vi "RBF Graph Test.vi"() -> ()   [LabVIEW 2021]
panel:
  in  "Weights":dbl[](array[numeric])
  in  "RBF":cluster{"STD":dbl, "Number":i32}
  out "XY Graph":cluster{dbl[], dbl[]}[](graph)
  in  "x":cluster{"Number":i32, "x_0":dbl, "x_f":dbl}
  out "x":dbl[][](array[numeric])
  out "RBF Centers":dbl[][](array[numeric])
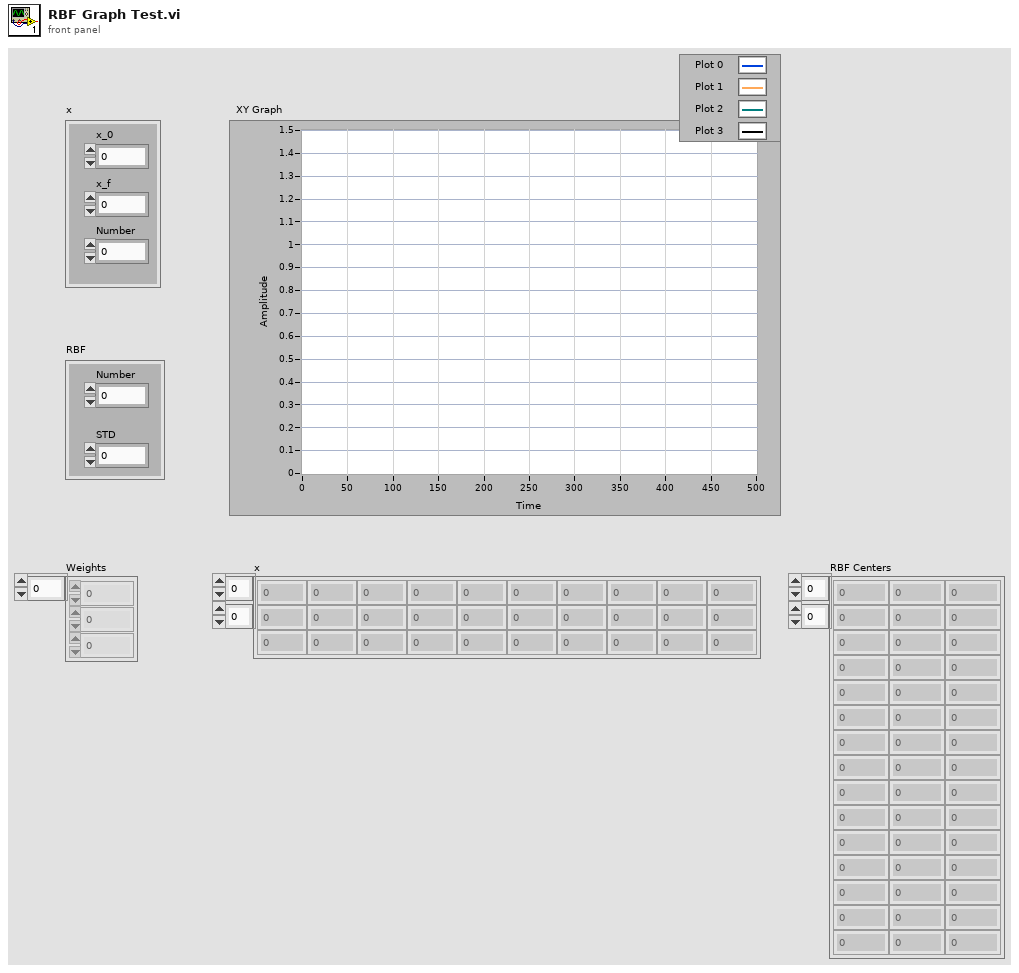
[diagram p1: front panel]
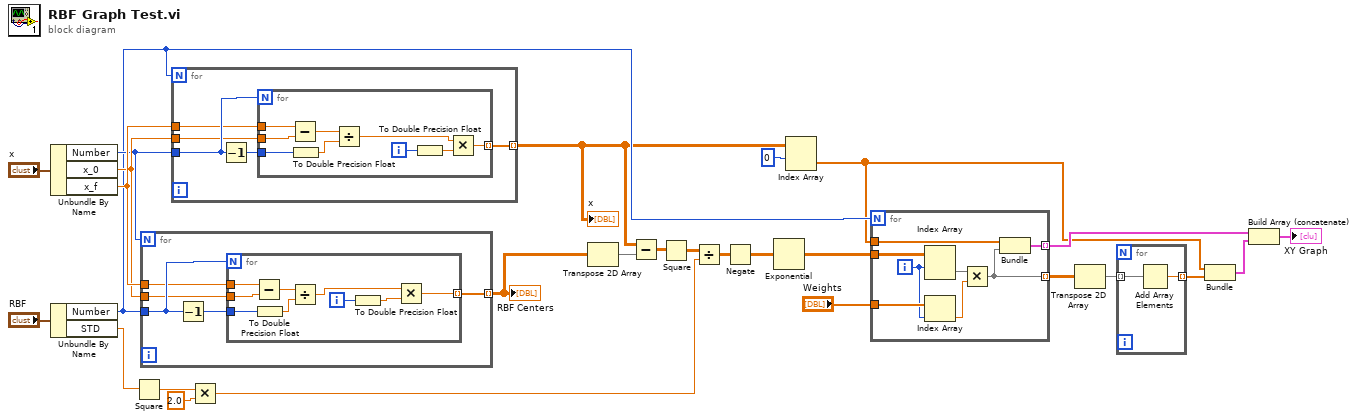
[diagram p0: block diagram]
diagram:
  n1 = Unbundle By Name("x") -> ("Number"=w15:i32, "x_0"=w17:dbl, "x_f"=w18:dbl)
  n2 = Unbundle By Name("RBF") -> ("Number"=w11:i32, "STD"=w16:dbl)
  n3 = Square(x=w16) -> (x^2=w25:dbl)
  n4 = for {
    N: w15 -> [_]
    tunnel: [w31] -> w13 mode=indexing
    tunnel: w11 -> [w30]
    tunnel: w18 -> [w29]
    tunnel: w17 -> [w28]
    n5 = Decrement(x=w30) -> (x-1=w32:i32)
    n6 = for {
      N: w30 -> [_]
      tunnel: w29 -> [w41]
      tunnel: w28 -> [w39]
      tunnel: [w40] -> w31 mode=indexing
      tunnel: w32 -> [w36]
      i -> [w34]
      n7 = Subtract(x=w41, y=w39) -> (x-y=w38:dbl)
      n8 = To Double Precision Float(number=w36) -> (double precision float=w35:dbl)
      n9 = Divide(x=w38, y=w35) -> (x/y=w37:dbl)
      n10 = To Double Precision Float(number=w34) -> (double precision float=w33:dbl)
      n11 = Multiply(x=w37, y=w33) -> (x*y=w40:dbl)
    }
  }
  "RBF Centers" <- w13
  n12 = for {
    N: w11 -> [_]
    tunnel: [w45] -> w5 mode=indexing
    tunnel: w15 -> [w44]
    tunnel: w18 -> [w43]
    tunnel: w17 -> [w42]
    n13 = Decrement(x=w44) -> (x-1=w46:i32)
    n14 = for {
      N: w44 -> [_]
      tunnel: w43 -> [w55]
      tunnel: w42 -> [w53]
      tunnel: [w54] -> w45 mode=indexing
      tunnel: w46 -> [w50]
      i -> [w47]
      n15 = Subtract(x=w55, y=w53) -> (x-y=w52:dbl)
      n16 = To Double Precision Float(number=w50) -> (double precision float=w49:dbl)
      n17 = Divide(x=w52, y=w49) -> (x/y=w51:dbl)
      n18 = To Double Precision Float(number=w47) -> (double precision float=w48:dbl)
      n19 = Multiply(x=w51, y=w48) -> (x*y=w54:dbl)
    }
  }
  "x" <- w5
  n20 = Multiply(x=w25, y=2.0) -> (x*y=w24:dbl)
  n21 = Transpose 2D Array(2D array=w13) -> (transposed array=w12:dbl[][])
  n22 = Subtract(x=w5, y=w12) -> (x-y=w27:dbl[][])
  n23 = Square(x=w27) -> (x^2=w23:dbl[][])
  n24 = Divide(x=w23, y=w24) -> (x/y=w22:dbl[][])
  n25 = Negate(x=w22) -> (-x=w21:dbl[][])
  n26 = Exponential(1:w21) -> (0:w2:dbl[][])
  n27 = Index Array(array=w5, index (row)=0) -> (element=w3:dbl[])  [unwired: 1 in]
  n28 = for {
    N: w11 -> [_]
    tunnel: w2 -> [w63]
    tunnel: [w62] -> w8 mode=indexing
    tunnel: "Weights" -> [w61]
    tunnel: w3 -> [w57]
    tunnel: [w56] -> w1 mode=indexing
    i -> [w60]
    n29 = Index Array(array=w63, index (row)=w60) -> (element=w58:dbl[])  [unwired: 1 in]
    n30 = Index Array(array=w61, index=w60) -> (element=w59:dbl)
    n31 = Multiply(x=w58, y=w59) -> (x*y=w56:dbl[])
    n32 = Bundle(w57, w56) -> (w62:cluster{dbl[], dbl[]})  [unwired: 1 in]
  }
  n33 = Transpose 2D Array(2D array=w1) -> (transposed array=w10:dbl[][])
  n34 = for {
    tunnel: w10 -> [w65] mode=indexing
    tunnel: [w64] -> w9 mode=indexing
    n35 = Add Array Elements(numeric array=w65) -> (sum=w64:dbl)
  }
  n36 = Bundle(w3, w9) -> (w6:cluster{dbl[], dbl[]})  [unwired: 1 in]
  n37 = Build Array (concatenate)(w8, w6) -> (→"XY Graph":cluster{dbl[], dbl[]}[])
